vi "Update Function Variables.vi"(8 "error in (no error)":errorcluster, 10 "Variable Names":string[](array[string]), 11 "Structure Loop in":refnum<class "Structure Loop.lvclass">) -> (0 "error out":errorcluster, 3 "Structure Loop out":refnum<class "Structure Loop.lvclass">)   [LabVIEW 2016, in "Structure Loop.lvclass"]
uses:
  Structure Loop.lvclass
  E:/Repository/LabVIEW Script Language/source code/LSL components/functions/functionsbase/functionbase.lvclass
  functionsbase/functionbase.lvclass/functionbase.ctl
  functionsbase/functionbase.lvclass
  functionsbase/properties/Read Func Full String.vi
  functionsbase/properties/Read RT Variables.vi
  variables/RT Variables/RT Variables.lvclass
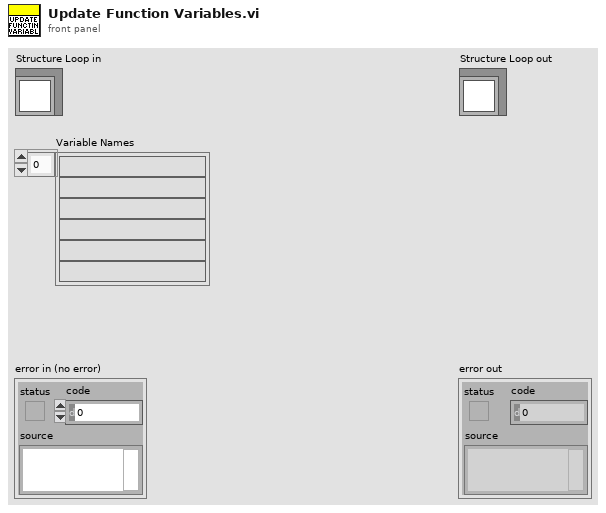
[diagram p1: front panel]
types:
  T1 = typedef "Datatype.ctl" = enum16{"Null", "Numeric", "String", "Bool", "Numeric 1D", "String 1D", "Bool 1D", "Numeric 2D", "String 2D", "Bool 2D", "Variant"}
  T2 = typedef "Valuetype.ctl" = enum16{"Value", "Variable", "Function"}
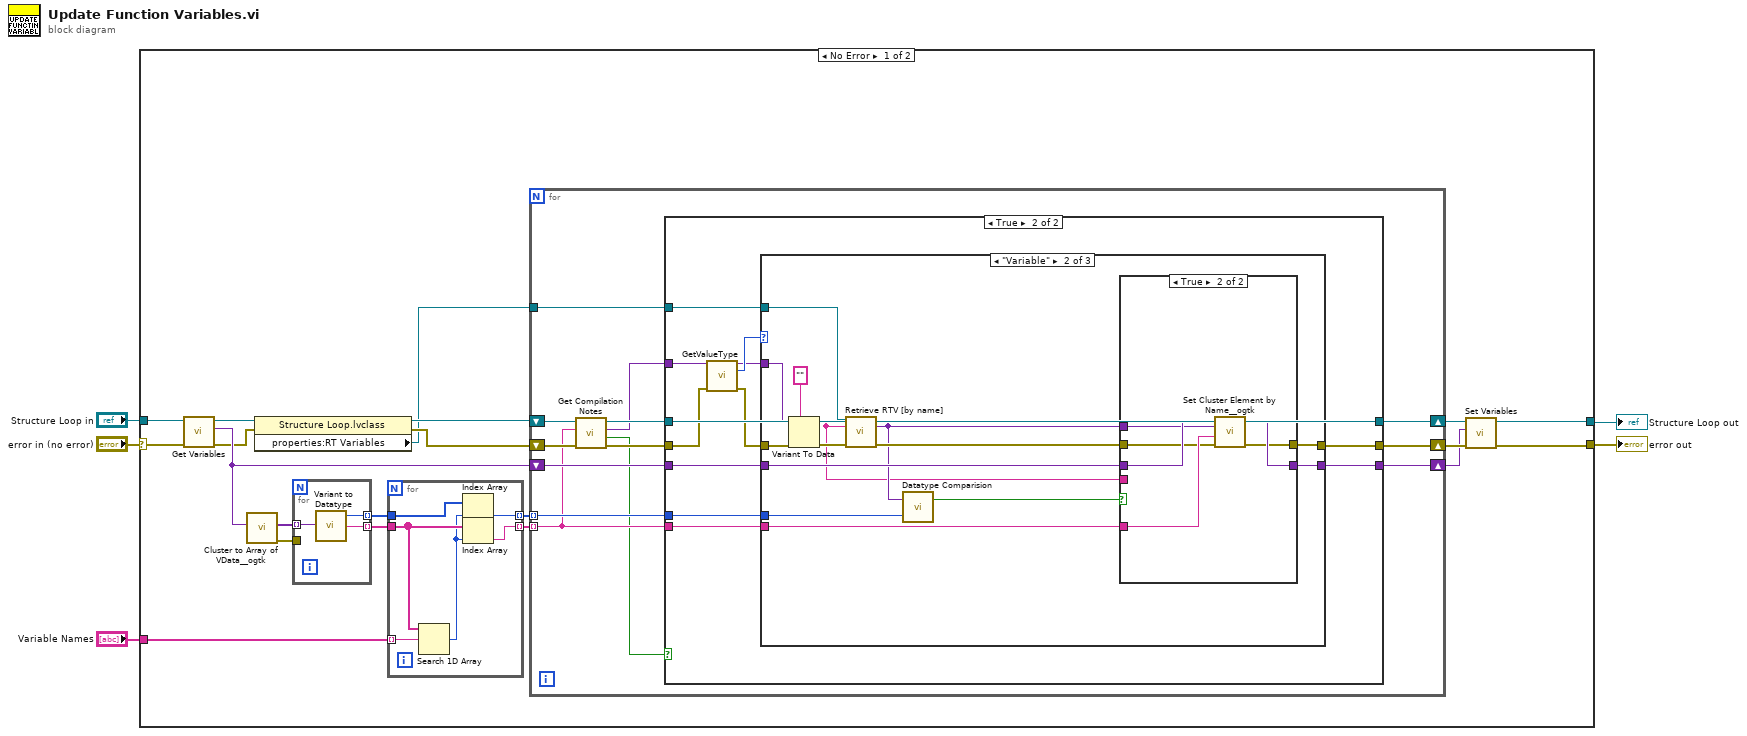
[diagram p0: block diagram]
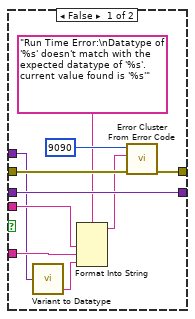
[diagram p4: hidden frame]
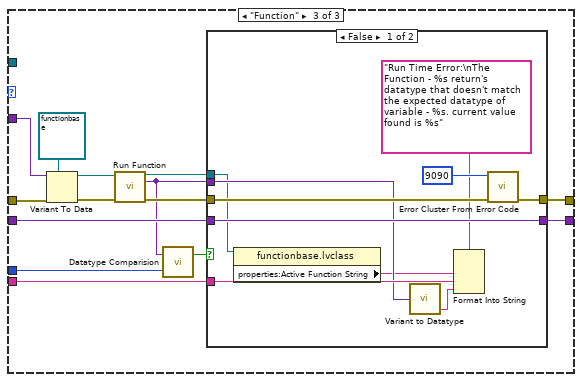
[diagram p5: hidden frame]
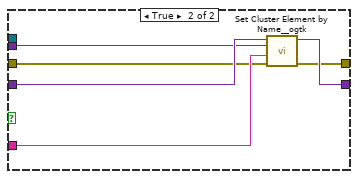
[diagram p6: hidden frame]
diagram:
  n1 = case shown="No Error" "error in (no error)" {
    selector: "error in (no error)" -> [w24 w126]
    tunnel: [w17 w126] -> w3
    tunnel: [w16 w125] -> w2
    tunnel: "Structure Loop in" -> [w23 w125]
    tunnel: "Variable Names" -> [w6 _]
    frame No Error {
      n2 = call-dynamic "Get Variables.vi"("error in (no error)"=w24, "For Loop in"=w23) -> ("error out"=w13:errorcluster, "Variables"=w21:variant, "For Loop out"=w15:refnum<class "Structure Loop.lvclass">)  [unwired: 7 in]
      n3 = call <userlib>:"Cluster to Array of VData__ogtk.vi"("Cluster"=w21) -> ("error out"=w22:errorcluster, "Array of VData"=w25:variant[])  [unwired: 9 in]
      n4 = property class="Structure Loop.lvclass"(reference=w15, error in=w13) -> (reference out=w14:refnum<class "Structure Loop.lvclass">, error out=w12:errorcluster, "properties:RT Variables"=w11:refnum<class "RT Variables.lvclass">)
      n5 = for {
        tunnel: w25 -> [w124] mode=indexing
        tunnel: [w123] -> w9 mode=indexing
        tunnel: [w122] -> w10 mode=indexing
        tunnel: w22 -> [_]
        n6 = call "Variant to Datatype.vi"("Variant"=w124) -> ("Name"=w122:string, "Datatype"=w123:T1)  [unwired: 2 in, 1 out]
      }
      n7 = for {
        tunnel: w6 -> [w31] mode=indexing
        tunnel: w10 -> [w30]
        tunnel: w9 -> [w29]
        tunnel: [w27] -> w8 mode=indexing
        tunnel: [w26] -> w7 mode=indexing
        n8 = Search 1D Array(1D array=w30, element=w31) -> (index of element=w28:i32)  [unwired: 1 in]
        n9 = Index Array(array=w29, index=w28) -> (element=w26:T1)
        n10 = Index Array(array=w30, index=w28) -> (element=w27:string)
      }
      n11 = for {
        shift-right: [w36] -> w20
        shift-left: w14 -> [w43]
        tunnel: w8 -> [w33] mode=indexing
        shift-right: [w41] -> w18
        shift-left: w21 -> [w42]
        shift-right: [w37] -> w19
        shift-left: w12 -> [w44]
        tunnel: w7 -> [w35] mode=indexing
        tunnel: w11 -> [w34]
        n12 = call "Get Compilation Notes.vi"("error in (no error)"=w44, "note key"=w33, "functionbase in"=w43) -> ("error out"=w39:errorcluster, "Found?"=w32:bool, "Notes"=w38:variant, "functionbase out"=w40:refnum<class "Structure Loop.lvclass">)  [unwired: 5 in]
        n13 = case shown="True" w32 {
          tunnel: w42 -> [w45 w53]
          tunnel: [w45 w54] -> w41
          tunnel: w40 -> [w47 w59]
          tunnel: w39 -> [w46 w57]
          tunnel: w38 -> [_ w58]
          tunnel: [w46 w52] -> w37
          tunnel: [w47 w59] -> w36
          tunnel: w35 -> [_ w50]
          tunnel: w33 -> [_ w49]
          tunnel: w34 -> [_ w48]
          frame False {
          }
          frame True {
            n14 = call "GetValueType.vi"("variant"=w58, "error in"=w57) -> ("variant out"=w55:variant, "Value Type"=w56:T2, "error out"=w51:errorcluster)  [unwired: 11 in]
            n15 = case shown="\"Variable\"" w56 {
              tunnel: w55 -> [_ w74 w104]
              tunnel: [w61 w70 w100] -> w54
              tunnel: w53 -> [w61 w71 w101]
              tunnel: [w60 w69 w97] -> w52
              tunnel: w51 -> [w60 w75 w105]
              tunnel: w50 -> [_ w66 w95]
              tunnel: w49 -> [_ w67 w99]
              tunnel: w48 -> [_ w64 _]
              frame "Value", Default {
              }
              frame "Variable" {
                n16 = Variant To Data(error in=w75, type="", Variant=w74) -> (data=w62:string, error out=w72:errorcluster)
                n17 = call-dynamic "Retrieve RTV [by name].vi"("RT Variables in"=w64, "RTV name"=w62, "error in (no error)"=w72) -> ("Data"=w63:variant, "error out"=w68:errorcluster)  [unwired: 8 in, 3 out]
                n18 = call "Datatype Comparision.vi"("Required Datatype"=w66, "Data"=w63) -> ("Equal?"=w65:bool)  [unwired: 1 out]
                n19 = case shown="True" w65 {
                  tunnel: w71 -> [w85 w91]
                  tunnel: [w85 w90] -> w70
                  tunnel: w63 -> [w77 w89]
                  tunnel: w67 -> [w78 w88]
                  tunnel: w68 -> [w84 w87]
                  tunnel: [w83 w86] -> w69
                  tunnel: w62 -> [w79 _]
                  frame False {
                    n20 = call "Variant to Datatype.vi"("Variant"=w77) -> ("Value"=w76:string)  [unwired: 2 in, 2 out]
                    n21 = Format Into String(format string="Run Time Error:\nDatatype of '%s' doesn't match with the expected datatype of '%s'. current value found is '%s'" ("error message (\"\")"), w79, w78, w76) -> (resulting string=w80:string)  [unwired: 2 in, 1 out]
                    n22 = call <vilib>:"Error Cluster From Error Code.vi"("error in (no error)"=w84, "error message (\"\")"=w80, "error code (0)"=9090) -> ("error out"=w83:errorcluster)  [unwired: 6 in]
                  }
                  frame True {
                    n23 = call <userlib>:"Set Cluster Element by Name__ogtk.vi"("error in (no error)"=w87, "Element Name (\"\": New Element Data Name)"=w88, "New Element Value"=w89, "Cluster"=w91) -> ("error out"=w86:errorcluster, "VCluster out"=w90:variant)  [unwired: 5 in, 1 out]
                  }
                }
              }
              frame "Function" {
                n24 = Variant To Data(error in=w105, type=refnum<class "functionbase.lvclass"> refnum ("functionbase.lvclass"), Variant=w104) -> (data=w93:refnum<class "functionbase.lvclass">, error out=w102:errorcluster)
                n25 = call-dynamic "Run Function.vi"("functionbase in"=w93, "error in (no error)"=w102) -> ("functionbase out"=w92:refnum<class "functionbase.lvclass">, "Return"=w96:variant, "error out"=w98:errorcluster)  [unwired: 11 in]
                n26 = call "Datatype Comparision.vi"("Required Datatype"=w95, "Data"=w96) -> ("Equal?"=w94:bool)  [unwired: 1 out]
                n27 = case shown="False" w94 {
                  tunnel: w101 -> [w115 w121]
                  tunnel: [w115 w120] -> w100
                  tunnel: w96 -> [w108 w119]
                  tunnel: w99 -> [w109 w118]
                  tunnel: w98 -> [w114 w117]
                  tunnel: [w113 w116] -> w97
                  tunnel: w92 -> [w107 _]
                  frame False {
                    n28 = property class="functionbase.lvclass"(reference=w107) -> ("properties:Active Function String"=w106:string)  [unwired: 1 in, 2 out]
                    n29 = call "Variant to Datatype.vi"("Variant"=w108) -> ("Value"=w111:string)  [unwired: 2 in, 2 out]
                    n30 = Format Into String(format string="Run Time Error:\nThe Function - %s return's datatype that doesn't match the expected datatype of variable - %s. current value found is %s" ("error message (\"\")"), w106, w109, w111) -> ()  [unwired: 2 in, 2 out]
                    n31 = call <vilib>:"Error Cluster From Error Code.vi"("error in (no error)"=w114, "error code (0)"=9090) -> ("error out"=w113:errorcluster)  [unwired: 7 in]
                  }
                  frame True {
                    n32 = call <userlib>:"Set Cluster Element by Name__ogtk.vi"("error in (no error)"=w117, "Element Name (\"\": New Element Data Name)"=w118, "New Element Value"=w119, "Cluster"=w121) -> ("error out"=w116:errorcluster, "VCluster out"=w120:variant)  [unwired: 5 in, 1 out]
                  }
                }
              }
            }
          }
        }
      }
      n33 = call-dynamic "Set Variables.vi"("error in (no error)"=w19, "Variables"=w18, "For Loop in"=w20) -> ("error out"=w17:errorcluster, "For Loop out"=w16:refnum<class "Structure Loop.lvclass">)  [unwired: 7 in]
    }
    frame Error {
    }
  }
  "error out" <- w3
  "Structure Loop out" <- w2
